vi "Drive Stuff.vi"() -> ()   [LabVIEW 2016]
doc: "This VI is not intended to be used in robot code. This is a stand alone VI intended to demonstrate the different drive methods shown in DiabloV1 and DiabloV2.\n\nCreated by Team 4130 for use in the 2016-2017 FRC season"
panel:
  in  "X":bool
  in  "stop":bool
  in  "Speed incriment":dbl
  in  "Y":bool
  in  "B":bool
  in  "A":bool
  in  "Right Stick Y":dbl(slide) scale=-1.0..1.0
  in  "Left Trigger":dbl(slide) scale=0.0..1.0
  in  "Right Trigger":dbl(slide) scale=0.0..1.0
  in  "Left Sick Y":dbl(slide) scale=-1.0..1.0
  in  "Left Stick X":dbl(slide) min=-1.0 max=1.0 scale=-1.0..1.0
  out "Left Drive":dbl
  out "Right Drive":dbl
  in  "Drive Mode":u16(ring) items=["Tank Drive Stright Speed", "Tank Drive Stright", "Tank Drive Speed", "Tank Drive", "Arcade Race Stright Speed", "Arcade Race Stright", "Arcade Race Speed", "Arcade Race", "Arcade Joystick Stright Speed", "Arcade Joystick Stright", "Arcade Joystick Speed", "Arcade Joystick"]
  out "Speed":dbl
  in  "Drive Stright\nSensitivity":dbl
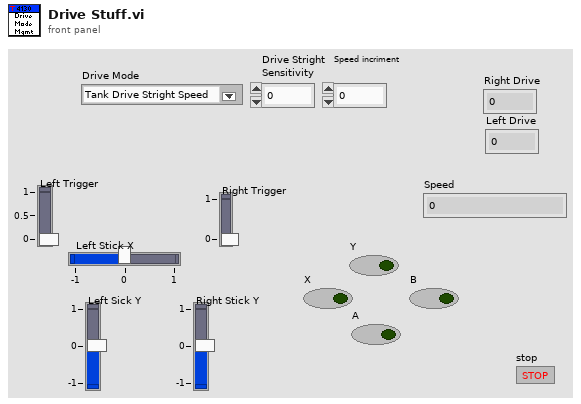
[diagram p1: front panel]
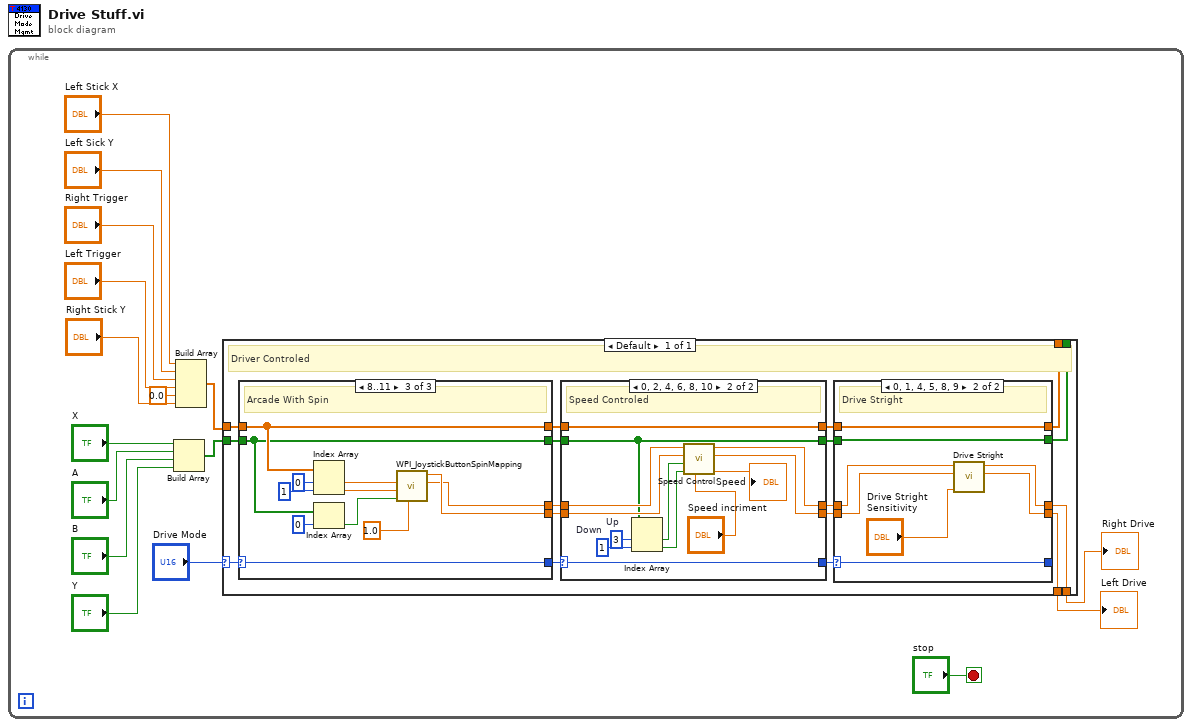
[diagram p0: block diagram]
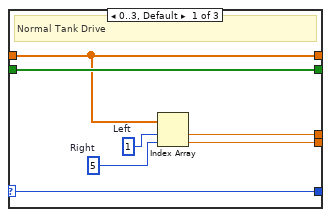
[diagram p4: hidden frame]
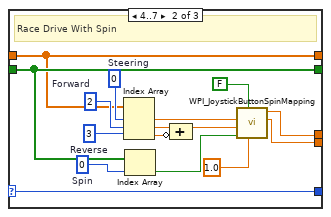
[diagram p5: hidden frame]
diagram:
  n1 = while {
    stop <- "stop" stop-if-true
    n2 = Build Array("X", "A", "B", "Y") -> (w9:bool[])
    n3 = Build Array("Left Stick X", "Left Sick Y", "Right Trigger", "Left Trigger", 0.0 ("element"), "Right Stick Y") -> (w14:dbl[])
    n4 = case shown="Default" "Drive Mode" {
      selector: "Drive Mode" -> [w31]
      tunnel: w14 -> [w33]
      tunnel: w9 -> [w32]
      tunnel: [w27] -> w16
      tunnel: [w24] -> w2
      tunnel: [w18] -> _
      tunnel: [w17] -> _
      frame Default {
        # "Driver Controled"
        n5 = case shown="8..11" w31 {
          selector: w31 -> [w65 w87 w96]
          tunnel: w33 -> [w66 w79 w97]
          tunnel: w32 -> [w67 w80 w89]
          tunnel: [w69 w77 w94] -> w30
          tunnel: [w68 w76 w95] -> w29
          tunnel: [w67 w80 w89] -> w28
          tunnel: [w66 w79 w97] -> w22
          tunnel: [w65 w87 w96] -> w20
          frame 0..3, Default {
            w70 = 5  # Right
            w71 = 1  # Left
            # "Normal Tank Drive"
            n6 = Index Array(array=w66, index #1=w71, index #2=w70) -> (element #1=w69:dbl, element #2=w68:dbl)
          }
          frame 4..7 {
            w78 = 3  # Reverse
            w82 = 0  # Spin
            w85 = 2  # Forward
            w86 = 0  # Steering
            # "Race Drive With Spin"
            n7 = Index Array(array=w79, index #1=w86, index #2=w85, index #3=w78) -> (element #1=w84:dbl, element #2=w74:dbl, element #3=w75:dbl)
            n8 = Index Array(array=w80, index=w82) -> (element=w81:bool)
            n9 = Compound Arithmetic op=ADD(w74, invert w75) -> (w73:dbl)
            n10 = call <vilib>:"WPI_JoystickButtonSpinMapping.vi"("Max Output"=1.0, "Square Inputs"=FALSE, "Spin?"=w81, "Y axis value"=w73, "X axis value"=w84) -> ("Right Motor Value"=w76:dbl, "Left Motor Value"=w77:dbl)  [unwired: 5 in]
          }
          frame 8..11 {
            # "Arcade With Spin"
            n11 = Index Array(array=w97, index #1=0 ("index"), index #2=1 ("index")) -> (element #1=w92:dbl, element #2=w93:dbl)
            n12 = Index Array(array=w89, index=0) -> (element=w88:bool)
            n13 = call <vilib>:"WPI_JoystickButtonSpinMapping.vi"("Max Output"=1.0, "Spin?"=w88, "Y axis value"=w93, "X axis value"=w92) -> ("Right Motor Value"=w94:dbl, "Left Motor Value"=w95:dbl)  [unwired: 6 in]
          }
        }
        n14 = case shown="0, 2, 4, 6, 8, 10" w20 {
          selector: w20 -> [w47 w54]
          tunnel: w30 -> [w51 w64]
          tunnel: w29 -> [w50 w63]
          tunnel: [w51 w62] -> w26
          tunnel: [w50 w61] -> w25
          tunnel: w28 -> [w48 w56]
          tunnel: [w49 w55] -> w23
          tunnel: w22 -> [w49 w55]
          tunnel: [w48 w56] -> w21
          tunnel: [w47 w54] -> w19
          frame Default {
            # "No Speed Limitation"
          }
          frame 0, 2, 4, 6, 8, 10 {
            w60 = 1  # Down
            w59 = 3  # Up
            # "Speed Controled"
            n15 = Index Array(array=w56, index #1=w59, index #2=w60) -> (element #1=w58:bool, element #2=w57:bool)
            n16 = call "Speed Control.vi"("Multiple"="Speed incriment", "Down"=w57, "Up"=w58, "Left Joystick"=w63, "Right Joystick"=w64) -> ("Speed"=→"Speed":dbl, "Left Motor"=w61:dbl, "Right Output"=w62:dbl)  [unwired: 4 in]
          }
        }
        n17 = case shown="0, 1, 4, 5, 8, 9" w19 {
          selector: w19 -> [w34 w44]
          tunnel: [w38 w41] -> w27
          tunnel: w26 -> [w38 w43]
          tunnel: w25 -> [w37 w42]
          tunnel: [w37 w40] -> w24
          tunnel: [w36 w46] -> w18
          tunnel: w23 -> [w36 w46]
          tunnel: [w35 w45] -> w17
          tunnel: w21 -> [w35 w45]
          tunnel: [w34 w44] -> _
          frame Default {
            # "Drive Direct"
          }
          frame 0, 1, 4, 5, 8, 9 {
            # "Drive Stright"
            n18 = call "Drive Stright.vi"("Dead Zone"="Drive Stright\nSensitivity", "Left Joystick"=w42, "Right Joystick"=w43) -> ("Left Drive Output"=w40:dbl, "Right Drive Output"=w41:dbl)  [unwired: 7 in]
          }
        }
      }
    }
    "Right Drive" <- w16
    "Left Drive" <- w2
  }
